vi "Lvi Subsystem Set Ctr Rate Mode.vi"(7 "GateLevel":u32, 8 "error in (no error)":errorcluster, 9 "DutyCycle":dbl, 10 "Frequency":dbl, 11 "TaskRef":i32) -> (0 "error out":errorcluster, 1 "function return":u32(ring), 2 "ActualFrequency":dbl, 3 "TaskRef out":i32)   [LabVIEW 2022 SP3, in "DtLvLink.lvlib"]
doc: "Calls directly into the entry points of the DLL of the Data Acq SDK to create one or more virtual channels, add them to a task, and configure the task with the specified settings to generate output pulses continuously at a specified frequency (in Hz) when the counter/timer is enabled (determined by the counter/timer's gate input signal). This VI is used by the higher-level VI, DtOLCreateTask."
uses:
  DtLvLink.lvlib
  <userlib>/LV-Link3/DtLvLink_64.dll
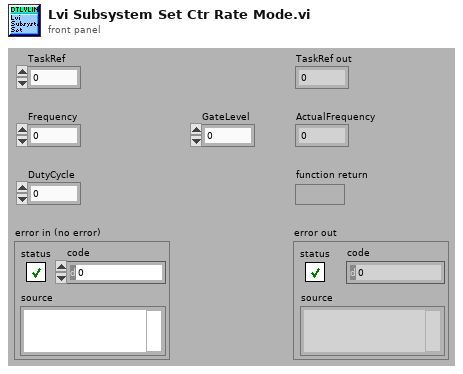
[diagram p1: front panel]
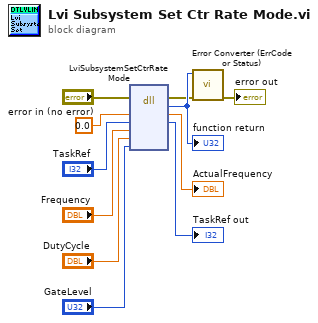
[diagram p0: block diagram]
diagram:
  n1 = dll-call lib="C:/Program Files/National Instruments/LabVIEW 2022/user.lib/LV-Link3/DtLvLink_64.*" fn="LviSubsystemSetCtrRateMode"(error in="error in (no error)", "ActualFrequency"=0.0, "TaskRef"="TaskRef", "Frequency"="Frequency", "DutyCycle"="DutyCycle", "GateLevel"="GateLevel") -> (error out=w2:errorcluster, w11:u32, "ActualFrequency"=→"ActualFrequency":dbl, "TaskRef"=→"TaskRef out":i32)  [unwired: 5 in, 1 out]
  "function return" <- w11
  n2 = call "Error Converter (ErrCode or Status).vi"("error in (no error)"=w2, "error code"=w11) -> ("error out"=→"error out":errorcluster)  [unwired: 9 in]
